vi "Get Exported DTC.vi"(8 "error in (no error)":errorcluster, 10 "DTCs GUID":string, 11 "Section Ref in":T1 format="%.0x") -> (0 "error out":errorcluster, 2 "DTC":T2, 3 "Section Ref out":T1 format="%.0x")   [LabVIEW 2015, in "Diagnostics Addon System Explorer.lvlib"]
uses:
  Diagnostics Addon System Explorer.lvlib
  Shared/Exported DTC Cluster.ctl
  <vilib>/Automotive Diagnostic Command Set/Diagnostic Protocols.llb/DTC Descriptor.ctl
  <vilib>/NI Veristand/Custom Device API/Custom Device Item Ref.ctl
  Shared/FG Action.ctl
  <vilib>/NI Veristand/Custom Device API/NI VeriStand - Get Item Property.vi
  <vilib>/NI Veristand/Custom Device API/Get Item Property (Variant).vi
  <vilib>/NI Veristand/Custom Device API/NI VeriStand - Set Item Property.vi
  <vilib>/NI Veristand/Custom Device API/Set Item Property (Variant).vi
  Shared/GUID Lookup.vi
  <vilib>/NI Veristand/Custom Device Tools/Custom Device Utility Library/NI VeriStand - Search for Item by GUID.vi
  Shared/Diagnostics Addon Shared.lvlib
  <vilib>/NI Veristand/Custom Device Tools/Custom Device Utility Library/Custom Device Utility Library.lvlib
  <vilib>/NI Veristand/Custom Device API/Custom Device API.lvlib
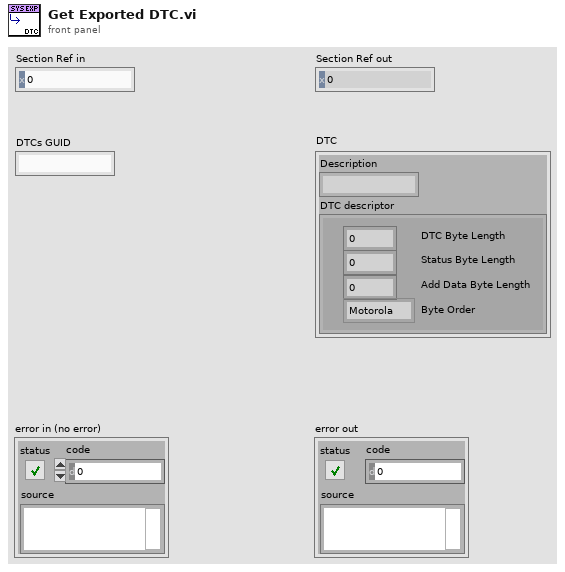
[diagram p1: front panel]
types:
  T1 = typedef "Custom Device API.lvlib/Custom Device Item Ref.ctl" = u64
  T2 = typedef "Diagnostics Addon Shared.lvlib/Exported DTC Cluster.ctl" = cluster{"Description":string, "DTC descriptor":T3}
  T3 = typedef "DTC Descriptor.ctl" = cluster{"DTC Byte Length":i32, "Status Byte Length":i32, "Add Data Byte Length":i32, "Byte Order":enum16{"Motorola", "Intel"}}
  T4 = typedef "Diagnostics Addon Shared.lvlib/FG Action.ctl" = enum16{"Get", "Set"}
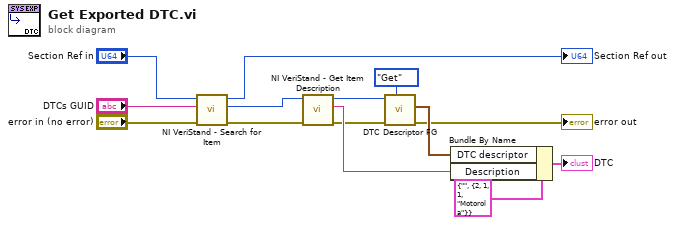
[diagram p0: block diagram]
diagram:
  n1 = call-poly <vilib>:"NI VeriStand - Search for Item.vi"("error in"="error in (no error)", "Item GUID"="DTCs GUID", "Section Ref in"="Section Ref in") -> ("error out"=w7:errorcluster, "Item Ref"=w8:T1, "Section Ref out"=→"Section Ref out":T1)  [unwired: 5 in, 1 out]
  n2 = call <vilib>:"NI VeriStand - Get Item Description.vi"("error in (no error)"=w7, "Item Ref in"=w8) -> ("error out"=w9:errorcluster, "Description"=w12:string, "Item Ref out"=w10:T1)  [unwired: 7 out]
  n3 = call "DTC Descriptor FG.vi"("Action"=FG_Action."Get", "error in (no error)"=w9, "Device Item Ref in"=w10) -> ("error out"=→"error out":errorcluster, "DTC descriptor"=w13:T3)  [unwired: 6 in, 1 out]
  n4 = Bundle By Name(cluster=T2 {"Description"="", "DTC descriptor"={"DTC Byte Length"=2, "Status Byte Length"=1, "Add Data Byte Length"=1, "Byte Order"=enum."Motorola"}}, "DTC descriptor"=w13, "Description"=w12) -> (→"DTC":T2)
